vi "Calculate Temperature Change-setup.vi"(11 "test case ID":string) -> (0 "Shutdown":bool, 1 "Time Interval (s)":dbl, 2 "Actual Temperature in deg C":dbl, 3 "Required Temperature deg C":dbl, 5 "Ramp Rate deg C/s":dbl)   [LabVIEW 2018]
doc: "The setup VI should be executed before the VI under test in the harness VI. In this VI you can prepare the environment and the inputs of the VI under test.\n\nSee the Help Document for more information. (<b>Help</b> > <b>IncQuery Labs</b> > <b>InstaCoverage</b> > <b>InstaCoverage Help...</b>)"
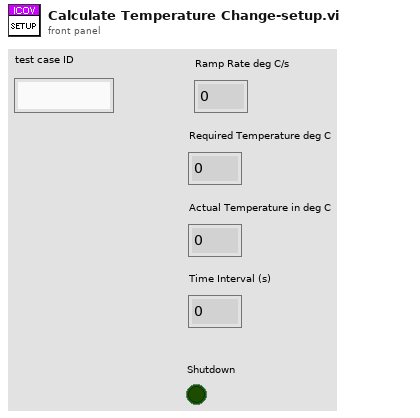
[diagram p1: front panel]
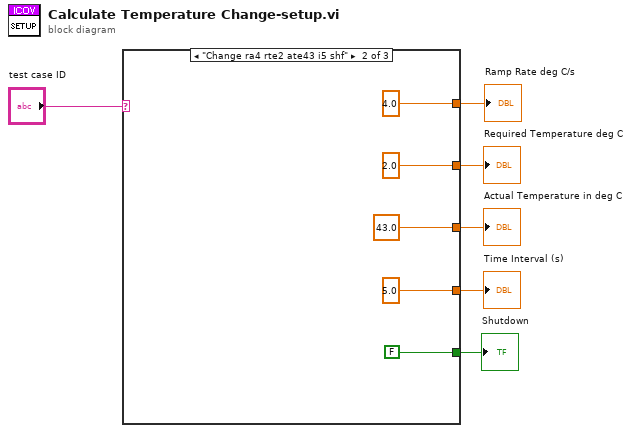
[diagram p0: block diagram]
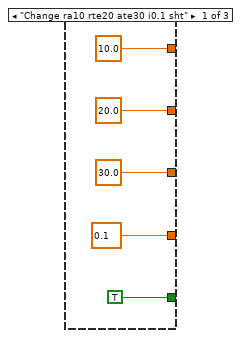
[diagram p2: hidden frame]
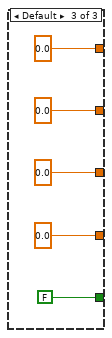
[diagram p3: hidden frame]
diagram:
  n1 = case shown="\"Change ra4 rte2 ate43 i5 shf\"" "test case ID" {
    tunnel: [10.0 4.0 0.0] -> w5
    tunnel: [30.0 43.0 0.0] -> w4
    tunnel: [0.1 5.0 0.0] -> w3
    tunnel: [TRUE FALSE FALSE] -> w2
    tunnel: [20.0 2.0 0.0] -> w1
    frame "Change ra10 rte20 ate30 i0.1 sht" {
    }
    frame "Change ra4 rte2 ate43 i5 shf" {
    }
    frame Default {
    }
  }
  "Ramp Rate deg C/s" <- w5
  "Actual Temperature in deg C" <- w4
  "Time Interval (s)" <- w3
  "Shutdown" <- w2
  "Required Temperature deg C" <- w1
